vi "DelayGeneratorGUI.vi"() -> ()   [LabVIEW 2009, in "DelayGenerator.lvlib"]
uses:
  DelayGenerator.lvlib
  Controls/Baseline.ctl
  Controls/SiteInformation.ctl
  Controls/StarAstrometricEntry.ctl
  Controls/DelayGeneratorState.ctl
panel:
  in  "+ Button":bool
  in  "- Button":bool
  in  "Step":dbl[unit] format="%.1g"
  out "Offset":dbl[unit] format="%.6g"
  out "State":T1
  in  "IDLE Button":bool
  in  "TRACK Button":bool
  in  "Star Astrometric Entry":T2={"catalog"="HIP", "starname"="ANTARES", "starnumber"=80763, "ra"=59364.46079999999, "dec"=-0.4613254627937262, "promora"=-1.5608487288736407e-15, "promodec"=-3.565679035153268e-15, "parallax"=8.144869842640205e-09, "radialvelocity"=0.0} {"dec" format="%.6g"; "ra" format="%.6g"}
  in  "Location":T3={"latitude"=0.34599908001030344, "longitude"=-2.713521559899555, "height"=4123.0, "temperature"=0.0, "pressure"=0.0} {"longitude" format="%_10g"; "latitude" format="%_10g"}
  in  "Baseline":T4={"East"=0.0, "North"=2.0, "Up"=0.0} {"Up" format="%.6g"; "North" format="%.6g"; "East" format="%.6g"}
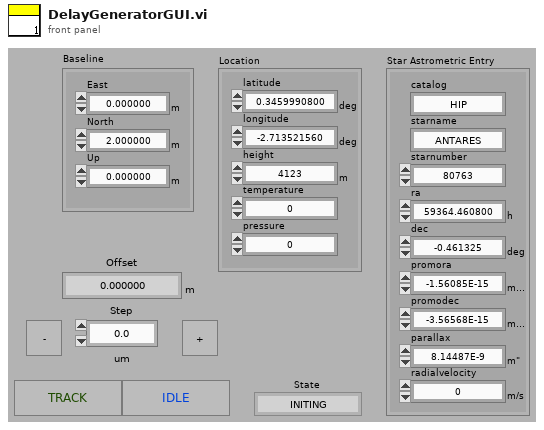
[diagram p1: front panel]
types:
  T1 = typedef "DelayGeneratorState.ctl" = enum16{"INITING", "IDLING", "TRACKING", "STOPPING"}
  T2 = typedef "StarAstrometricEntry.ctl" = cluster{"catalog":string, "starname":string, "starnumber":i32, "ra":dbl[unit], "dec":dbl[unit], "promora":dbl[unit], "promodec":dbl[unit], "parallax":dbl[unit], "radialvelocity":dbl[unit]}
  T3 = typedef "SiteInformation.ctl" = cluster{"latitude":dbl[unit], "longitude":dbl[unit], "height":dbl[unit], "temperature":dbl, "pressure":dbl}
  T4 = typedef "Baseline.ctl" = cluster{"East":dbl[unit], "North":dbl[unit], "Up":dbl[unit]}
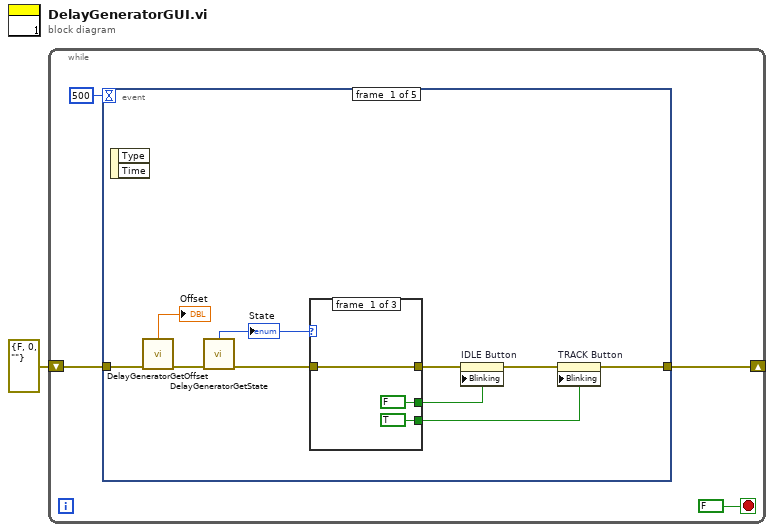
[diagram p0: block diagram]
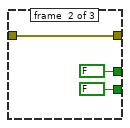
[diagram p2: hidden frame]
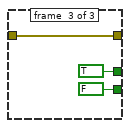
[diagram p3: hidden frame]
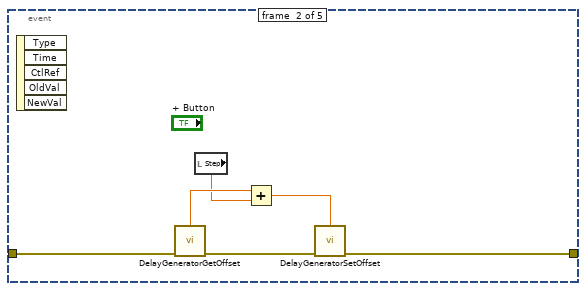
[diagram p4: hidden frame]
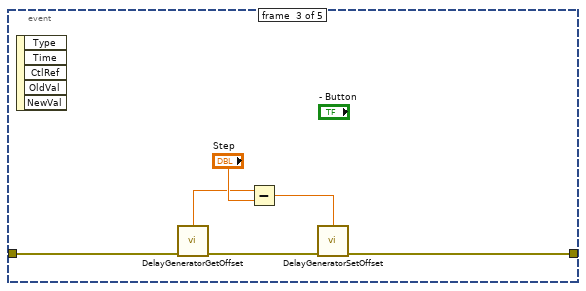
[diagram p5: hidden frame]
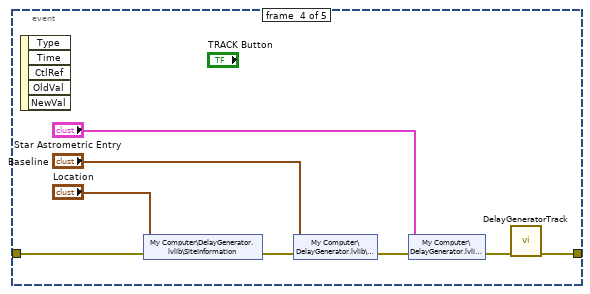
[diagram p6: hidden frame]
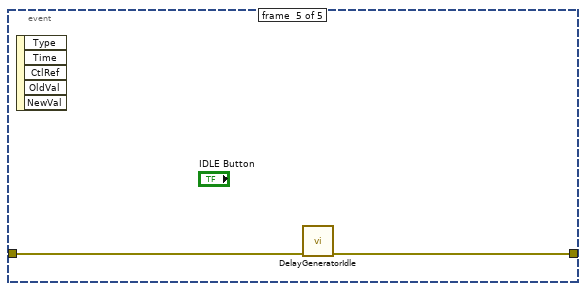
[diagram p7: hidden frame]
diagram:
  n1 = while {
    shift-right: [w5] -> _
    shift-left: errorcluster {"status"=FALSE, "code"=0, "source"=""} ("error out") -> [w4]
    stop <- FALSE stop-if-true
    n2 = event shown="[1] \"+ Button\": Value Change" {
      selector: _ -> [_ _ _ _ _]
      dyn-events: _ -> [_ _ _ _ _]
      timeout: 500 -> [_ _ _ _ _]
      tunnel: w4 -> [w8 w27 w36 w39 w46]
      tunnel: [w14 w26 w34 w37 w45] -> w5
      event #0 {
        n3 = event-data() -> ()  [unwired: 1 in, 2 out]
        n4 = call "DelayGeneratorGetOffset.vi"("error in (no error)"=w8) -> ("Offset"=→"Offset":dbl[unit], "error out"=w7:errorcluster)  [unwired: 7 in]
        n5 = call "DelayGeneratorGetState.vi"("error in (no error)"=w7) -> ("State"=w12:T1, "error out"=w13:errorcluster)  [unwired: 7 in]
        "State" <- w12
        n6 = case shown="Default" w12 {
          tunnel: w13 -> [w18 w21 w24]
          tunnel: [w18 w21 w24] -> w11
          tunnel: [FALSE FALSE TRUE] -> w10
          tunnel: [TRUE FALSE FALSE] -> w9
          frame #0 {
          }
          frame #1 {
          }
          frame #2 {
          }
        }
        n7 = property on="IDLE Button" class="Bool"(error in=w11, "Blinking"=w10) -> (error out=w15:errorcluster)  [unwired: 1 in, 1 out]
        n8 = property on="TRACK Button" class="Bool"(error in=w15, "Blinking"=w9) -> (error out=w14:errorcluster)  [unwired: 1 in, 1 out]
      }
      event #1 {
        n9 = event-data() -> ()  [unwired: 1 in, 5 out]
        n10 = call "DelayGeneratorGetOffset.vi"("error in (no error)"=w27) -> ("Offset"=w29:dbl[unit], "error out"=w30:errorcluster)  [unwired: 7 in]
        n11 = local read "Step"() -> (w25:dbl[unit])
        n12 = Add(x=w29, y=w25) -> (x+y=w28:dbl[unit])
        n13 = call "DelayGeneratorSetOffset.vi"("Offset"=w28, "error in (no error)"=w30) -> ("error out"=w26:errorcluster)  [unwired: 7 in]
      }
      event #2 {
        n14 = event-data() -> ()  [unwired: 1 in, 5 out]
        n15 = call "DelayGeneratorGetOffset.vi"("error in (no error)"=w36) -> ("Offset"=w32:dbl[unit], "error out"=w35:errorcluster)  [unwired: 7 in]
        n16 = Subtract(x=w32, y="Step") -> (x-y=w31:dbl[unit])
        n17 = call "DelayGeneratorSetOffset.vi"("Offset"=w31, "error in (no error)"=w35) -> ("error out"=w34:errorcluster)  [unwired: 7 in]
      }
      event #3 {
        n18 = event-data() -> ()  [unwired: 1 in, 5 out]
        n19 = shared-variable "My Computer\\DelayGenerator.lvlib\\SiteInformation"("Location", error in=w39) -> (error out=w43:errorcluster)
        n20 = shared-variable "My Computer\\DelayGenerator.lvlib\\Baseline"("Baseline", error in=w43) -> (error out=w41:errorcluster)
        n21 = shared-variable "My Computer\\DelayGenerator.lvlib\\Target"("Star Astrometric Entry", error in=w41) -> (error out=w38:errorcluster)
        n22 = call "DelayGeneratorTrack.vi"("error in (no error)"=w38) -> ("error out"=w37:errorcluster)  [unwired: 10 in]
      }
      event #4 {
        n23 = event-data() -> ()  [unwired: 1 in, 5 out]
        n24 = call "DelayGeneratorIdle.vi"("error in (no error)"=w46) -> ("error out"=w45:errorcluster)  [unwired: 10 in]
      }
    }
  }
